vi "DelayTableLoad.vi"(7 "Daxsonics Name":T1=enum."New2021", 9 "PRI (ns)":i32=25000, 10 "Delay Table (ns)":i32[][](array[numeric]), 11 "VISA Refnum in":refnum<visa-resource-name>) -> ()   [LabVIEW 2022 SP3]
uses:
  Daxsonics_Pulsers.ctl
panel:
  # "-1 delay means element off for xmit"
  # "Columns are element #"
  # "Rows are\nxmit \nevent"
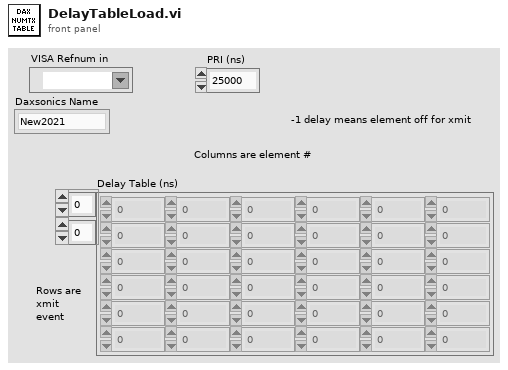
[diagram p1: front panel]
types:
  T1 = typedef "Daxsonics_Pulsers.ctl" = enum16{"BP1", "BP2_A", "BP2_B", "10ERS8", "New2021"}
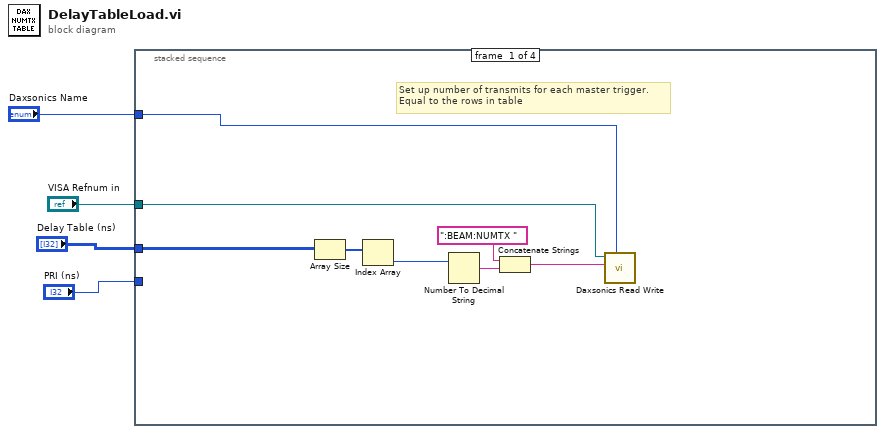
[diagram p0: block diagram]
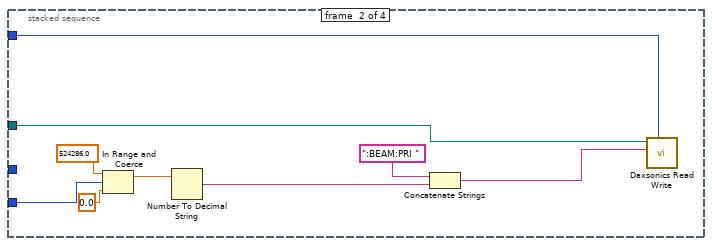
[diagram p2: hidden frame]
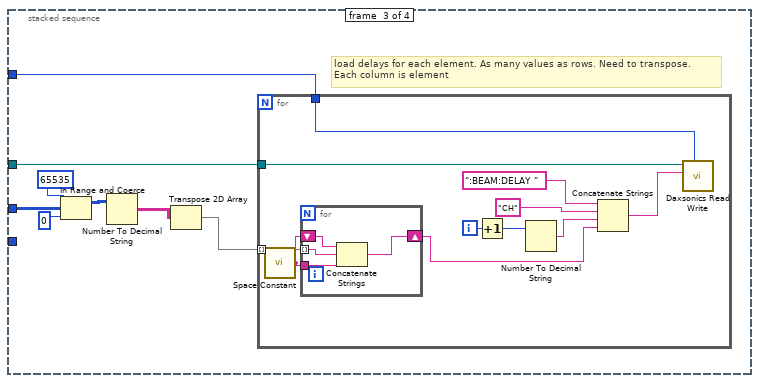
[diagram p3: hidden frame]
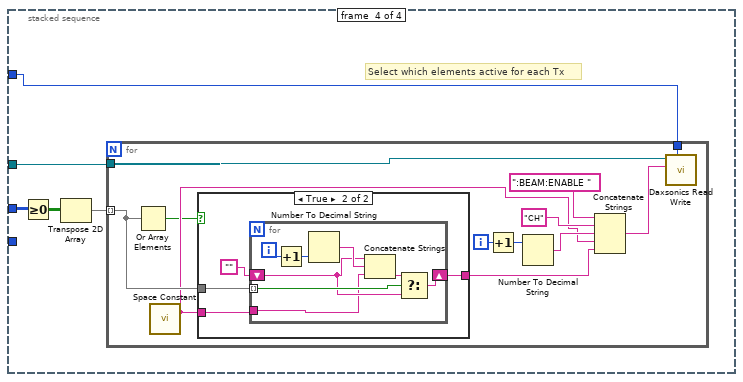
[diagram p4: hidden frame]
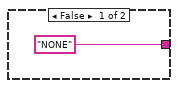
[diagram p5: hidden frame]
diagram:
  n1 = stacked-sequence {
    tunnel: "VISA Refnum in" -> [w9 w18 w27 w47]
    tunnel: "Delay Table (ns)" -> [w7 _ w26 w48]
    tunnel: "PRI (ns)" -> [_ w16 _ _]
    tunnel: "Daxsonics Name" -> [w5 w13 w22 w45]
    frame #0 {
      # "Set up number of transmits for each master trigger.\nEqual to the rows in table"
      n2 = Array Size(array=w7) -> (size(s)=w8:i32[])
      n3 = Index Array(array=w8) -> (element=w6:i32)  [unwired: 1 in]
      n4 = Number To Decimal String(number=w6) -> (decimal integer string=w11:string)  [unwired: 1 in]
      n5 = Concatenate Strings(":BEAM:NUMTX " ("string"), w11) -> (w10:string)
      n6 = call "Daxsonics Read Write.vi"("Daxsonics Name"=w5, "write buffer"=w10, "VISA resource name"=w9) -> ()  [unwired: 6 in, 3 out]
    }
    frame #1 {
      n7 = In Range and Coerce(upper limit=524286.0, x=w16, lower limit=0.0) -> (coerced(x)=w14:dbl)  [unwired: 1 out]
      n8 = Number To Decimal String(number=w14) -> (decimal integer string=w21:string)  [unwired: 1 in]
      n9 = Concatenate Strings(":BEAM:PRI " ("string"), w21) -> (w20:string)
      n10 = call "Daxsonics Read Write.vi"("Daxsonics Name"=w13, "write buffer"=w20, "VISA resource name"=w18) -> ()  [unwired: 6 in, 3 out]
    }
    frame #2 {
      # "load delays for each element. As many values as rows. Need to transpose.\nEach column is element"
      n11 = In Range and Coerce(upper limit=65535, x=w26, lower limit=0) -> (coerced(x)=w23:i32[][])  [unwired: 1 out]
      n12 = Number To Decimal String(number=w23) -> (decimal integer string=w29:string[][])  [unwired: 1 in]
      n13 = Transpose 2D Array(2D array=w29) -> (transposed array=w28:string[][])
      n14 = for {
        tunnel: w28 -> [w40] mode=indexing
        tunnel: w27 -> [w32]
        tunnel: w22 -> [w30]
        i -> [w38]
        n15 = call <vilib>:"Space Constant.vi"() -> ("String"=w33:string)
        n16 = for {
          tunnel: w40 -> [w44] mode=indexing
          shift-right: [w42] -> w35
          shift-left: w33 -> [w43]
          tunnel: w33 -> [w41]
          n17 = Concatenate Strings(w43, w44, w41) -> (w42:string)
        }
        n18 = Increment(x=w38) -> (x+1=w31:i32)
        n19 = Number To Decimal String(number=w31) -> (decimal integer string=w37:string)  [unwired: 1 in]
        n20 = Concatenate Strings(":BEAM:DELAY " ("string"), "CH", w37, w35) -> (w34:string)
        n21 = call "Daxsonics Read Write.vi"("Daxsonics Name"=w30, "write buffer"=w34, "VISA resource name"=w32) -> ()  [unwired: 6 in, 3 out]
      }
    }
    frame #3 {
      # "Select which elements active for each Tx"
      n22 = Greater Or Equal To 0?(x=w48) -> (x >= 0?=w49:bool[][])
      n23 = Transpose 2D Array(2D array=w49) -> (transposed array=w46:bool[][])
      n24 = for {
        tunnel: w47 -> [w57]
        tunnel: w46 -> [w53] mode=indexing
        tunnel: w45 -> [w50]
        i -> [w61]
        n25 = Or Array Elements(Boolean array=w53) -> (logical OR=w51:bool)
        n26 = call <vilib>:"Space Constant.vi"() -> ("String"=w52:string)
        n27 = case shown="True" w51 {
          tunnel: ["NONE" w66] -> w54
          tunnel: w53 -> [_ w64]
          tunnel: w52 -> [_ w63]
          frame False {
          }
          frame True {
            n28 = for {
              tunnel: w64 -> [w71] mode=indexing
              shift-right: [w73] -> w66
              shift-left: "" -> [w68]
              tunnel: w63 -> [w67]
              i -> [w74]
              n29 = Increment(x=w74) -> (x+1=w70:i32)
              n30 = Number To Decimal String(number=w70) -> (decimal integer string=w69:string)  [unwired: 1 in]
              n31 = Concatenate Strings(w68, w69, w67) -> (w72:string)
              n32 = Select(t=w72, s=w71, f=w68) -> (s? t:f=w73:string)
            }
          }
        }
        n33 = Increment(x=w61) -> (x+1=w55:i32)
        n34 = Number To Decimal String(number=w55) -> (decimal integer string=w60:string)  [unwired: 1 in]
        n35 = Concatenate Strings(":BEAM:ENABLE " ("string"), "CH", w60, w52, w54) -> (w58:string)
        n36 = call "Daxsonics Read Write.vi"("Daxsonics Name"=w50, "write buffer"=w58, "VISA resource name"=w57) -> ()  [unwired: 6 in, 3 out]
      }
    }
  }
